vi "GFL_Get_Single_Fault_Snapshot.vi"(0 "GEA2 Reference In":refnum<k24>, 5 "Standalone?":bool, 7 "Snapshot Selection":T2, 11 "Error In":errorcluster) -> (4 "GEA2 Reference Out":refnum<k24>, 6 "Fault Snapshots":T1, 15 "Error Out":errorcluster)   [LabVIEW 2016]
uses:
  subVIs/Snap_Selection.ctl
  C:/Automation/DLLs/PC Dot Net/GeaCommunication.dll
  subVIs/Snap_Input.ctl
  Common/LabVIEW GEA2 Toolkit/LabVIEW_GEA2_Toolkit.lvlibp/type defs/Source_Destination.ctl
  Common/LabVIEW GEA2 Toolkit/LabVIEW_GEA2_Toolkit.lvlibp/type defs/ERD Read Data In.ctl
  Common/LabVIEW GEA2 Toolkit/LabVIEW_GEA2_Toolkit.lvlibp/type defs/Data Type.ctl
  Common/LabVIEW GEA2 Toolkit/LabVIEW_GEA2_Toolkit.lvlibp
panel:
  out "ERD Number":string
  out "ERD Data":string
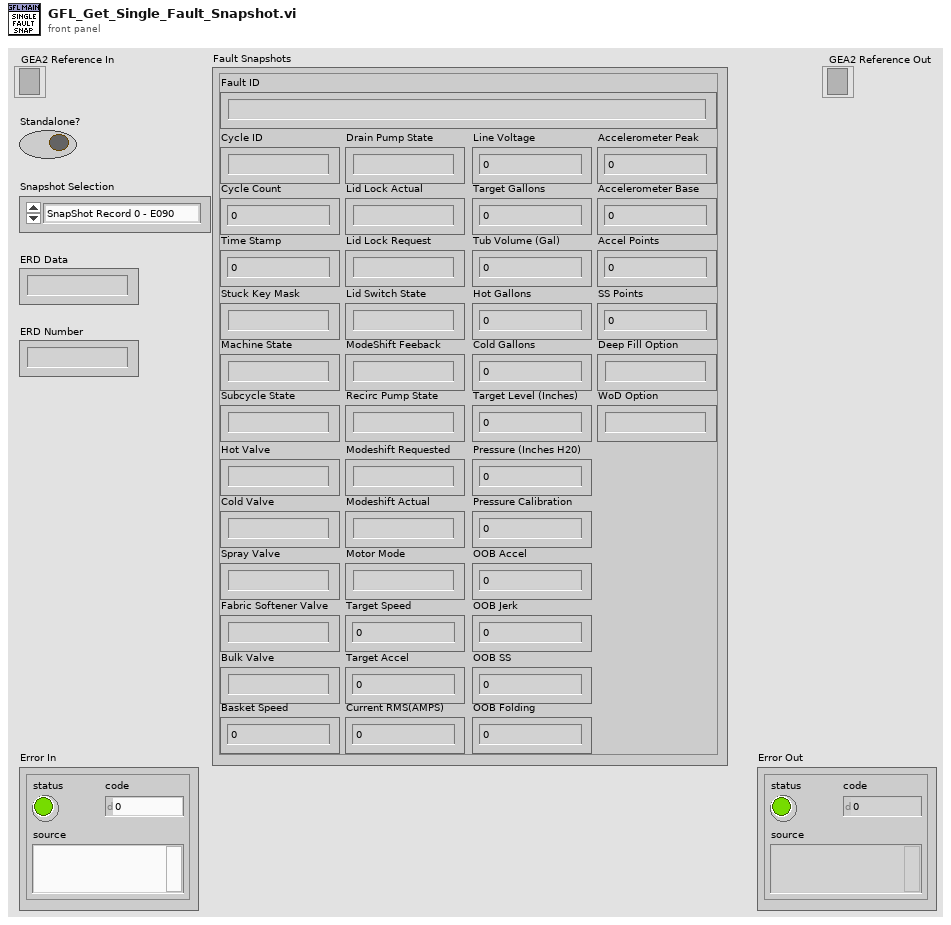
[diagram p1: front panel]
types:
  T1 = typedef "Snap_Input.ctl" = cluster{"Fault ID":string, "Cycle Count":u32, "Cycle ID":string, "Time Stamp":u32, "Stuck Key Mask":string, "Machine State":string, "Subcycle State":string, "Hot Valve":string, "Cold Valve":string, "Spray Valve":string, "Fabric Softener Valve":string, "Bulk Valve":string, "Drain Pump State":string, "Lid Lock Actual":string, "Lid Lock Request":string, "Lid Switch State":string, "ModeShift Feeback":string, "Recirc Pump State":string, "Modeshift Requested":string, "Modeshift Actual":string, "Motor Mode":string, "Target Speed":u16, "Target Accel":u16, "Current RMS(AMPS)":dbl, "Line Voltage":dbl, "Target Gallons":dbl, "Tub Volume (Gal)":dbl, "Hot Gallons":dbl, "Cold Gallons":dbl, "Target Level (Inches)":dbl, "Pressure (Inches H20) ":dbl, "Pressure Calibration":dbl, "OOB Accel":i32, "OOB Jerk":i32, "OOB SS":i32, "OOB Folding":i32, "Accelerometer Peak":i16, "Accelerometer Base":i16, "Accel Points":u8, "SS Points":u8, "Deep Fill Option":string, "WoD Option":string, "Basket Speed":u16}
  T2 = typedef "Snap_Selection.ctl" = enum16{"SnapShot Record 0 - E090", "Snapshot Record 1 - E091", "Snapshot Record 2 - E092"}
  T3 = typedef "LabVIEW_GEA2_Toolkit.lvlibp/Source_Destination.ctl" = cluster{"Source":u8, "Destination":u8}
  T4 = typedef "LabVIEW_GEA2_Toolkit.lvlibp/ERD Read Data In.ctl" = cluster{"ERD Number":u16, "Data Type":T5}
  T5 = typedef "LabVIEW_GEA2_Toolkit.lvlibp/Data Type.ctl" = enum16{"string", "boolean", "uint8_t", "uint16_t", "uint32_t", "uint64_t", "int8_t", "int16_t", "int32_t", "int64_t"}
  T6 = typedef "LabVIEW_GEA2_Toolkit.lvlibp/ERD Read Data Out.ctl" = cluster{"ERD Number":u16, "Data":string}
  T7 = cluster{"ERD Data Out[0]":T6, "ERD Data Out[1]":T6, "ERD Data Out[2]":T6, "ERD Data Out[3]":T6, "ERD Data Out[4]":T6, "ERD Data Out[5]":T6, "ERD Data Out[6]":T6, "ERD Data Out[7]":T6, "ERD Data Out[8]":T6}
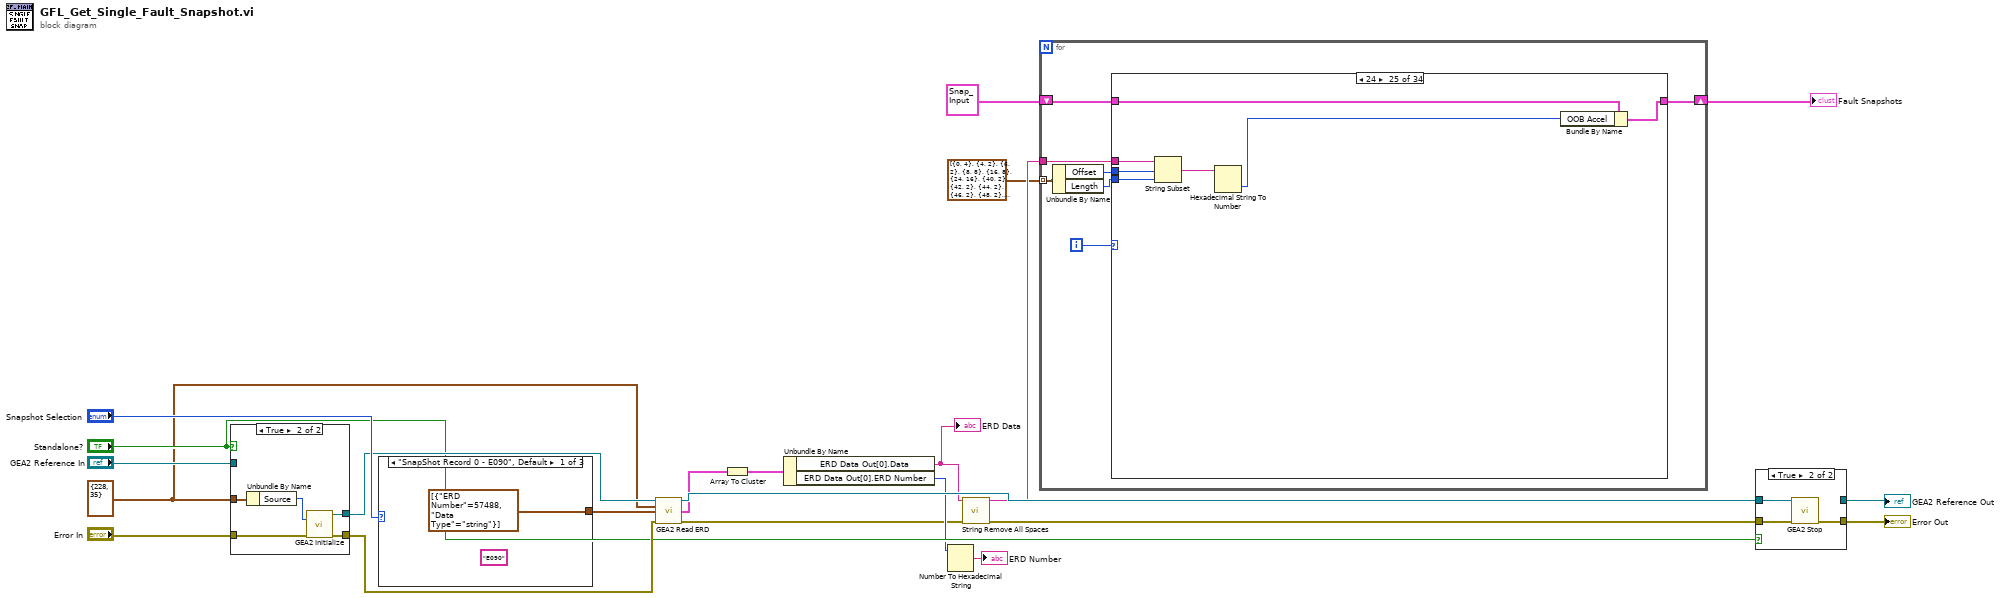
[diagram p0: block diagram]
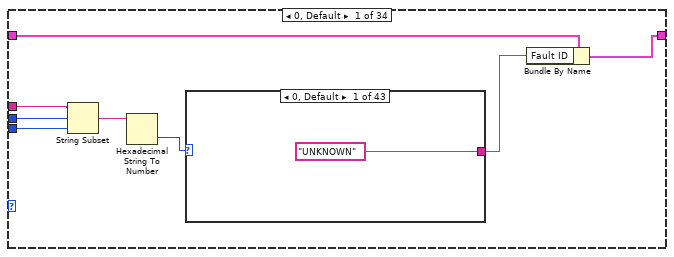
[diagram p2: hidden frame]
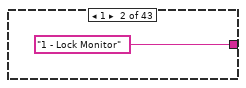
[diagram p3: hidden frame]
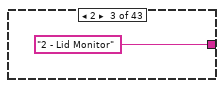
[diagram p4: hidden frame]
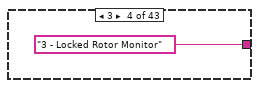
[diagram p5: hidden frame]
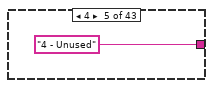
[diagram p6: hidden frame]
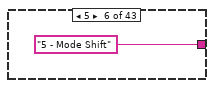
[diagram p7: hidden frame]
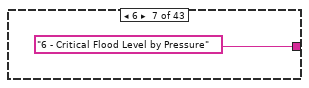
[diagram p8: hidden frame]
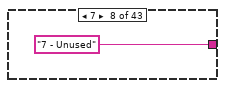
[diagram p9: hidden frame]
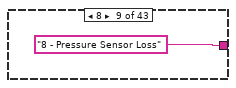
[diagram p10: hidden frame]
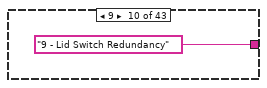
[diagram p11: hidden frame]
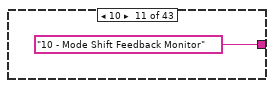
[diagram p12: hidden frame]
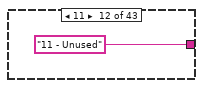
[diagram p13: hidden frame]
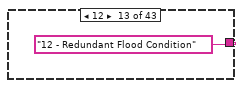
[diagram p14: hidden frame]
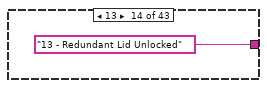
[diagram p15: hidden frame]
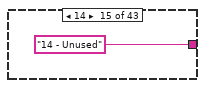
[diagram p16: hidden frame]
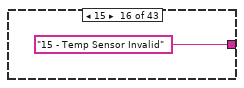
[diagram p17: hidden frame]
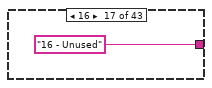
[diagram p18: hidden frame]
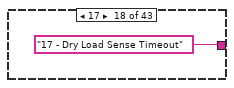
[diagram p19: hidden frame]
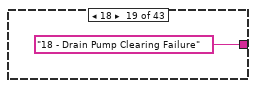
[diagram p20: hidden frame]
diagram:
  w13 = T3 {"Source"=228, "Destination"=35} ("GEA Inputs")
  n1 = case shown="True" "Standalone?" {
    tunnel: "Error In" -> [w23 w29]
    tunnel: [w23 w28] -> w17
    tunnel: "GEA2 Reference In" -> [w24 _]
    tunnel: [w24 w27] -> w18
    tunnel: w13 -> [_ w25]
    frame False {
    }
    frame True {
      n2 = Unbundle By Name(w25) -> ("Source"=w26:u8)
      n3 = call "GEA2 Initialize.vi"("Source Address"=w26, "error in"=w29) -> ("GEA2 Reference Out"=w27:refnum<k24>, "error out"=w28:errorcluster)  [unwired: 11 in, 1 out]
    }
  }
  n4 = case shown="\"SnapShot Record 0 - E090\", Default" "Snapshot Selection" {
    tunnel: [T4[] [{"ERD Number"=57488, "Data Type"=enum."string"}] ("Read ERD List") T4[] [{"ERD Number"=57489, "Data Type"=enum."string"}] ("Read ERD List") T4[] [{"ERD Number"=57490, "Data Type"=enum."string"}] ("Read ERD List")] -> w21
    frame "SnapShot Record 0 - E090", Default {
      (unwired) "E090"
    }
    frame "Snapshot Record 1 - E091" {
      (unwired) "E091"
    }
    frame "Snapshot Record 2 - E092" {
      (unwired) "E092"
    }
  }
  n5 = call "GEA2 Read ERD.vi"("GEA2 Reference In"=w18, "GEA Inputs"=w13, "Read ERD List"=w21, "Error In"=w17) -> ("GEA2 Reference Out"=w16:refnum<k24>, "ERD Data Out"=w12:T6[], "Error Out"=w7:errorcluster)  [unwired: 8 in, 1 out]
  n6 = Array To Cluster(array=w12) -> (cluster=w11:T7)
  n7 = Unbundle By Name(w11) -> ("ERD Data Out[0].Data"=w8:string, "ERD Data Out[0].ERD Number"=w10:u16)
  "ERD Data" <- w8
  n8 = Number To Hexadecimal String(2:w10) -> (0:→"ERD Number":string)  [unwired: 1 in]
  n9 = call "String Remove All Spaces.vi"("Input String"=w8, "error in (no error)"=w7) -> ("Spaces Removed"=w4:string, "error out"=w6:errorcluster)  [unwired: 12 in]
  n10 = for {
    tunnel: w4 -> [w39]
    shift-right: [w37] -> w1
    shift-left: T1 {"Fault ID"="", "Cycle Count"=0, "Cycle ID"="", "Time Stamp"=0, "Stuck Key Mask"="", "Machine State"="", "Subcycle State"="", "Hot Valve"="", "Cold Valve"="", "Spray Valve"="", "Fabric Softener Valve"="", "Bulk Valve"="", "Drain Pump State"="", "Lid Lock Actual"="", "Lid Lock Request"="", "Lid Switch State"="", "ModeShift Feeback"="", "Recirc Pump State"="", "Modeshift Requested"="", "Modeshift Actual"="", "Motor Mode"="", "Target Speed"=0, "Target Accel"=0, "Current RMS(AMPS)"=0.0, "Line Voltage"=0.0, "Target Gallons"=0.0, "Tub Volume (Gal)"=0.0, "Hot Gallons"=0.0, "Cold Gallons"=0.0, "Target Level (Inches)"=0.0, "Pressure (Inches H20) "=0.0, "Pressure Calibration"=0.0, "OOB Accel"=0, "OOB Jerk"=0, "OOB SS"=0, "OOB Folding"=0, "Accelerometer Peak"=0, "Accelerometer Base"=0, "Accel Points"=0, "SS Points"=0, "Deep Fill Option"="", "WoD Option"="", "Basket Speed"=0} ("input cluster") -> [w38]
    tunnel: cluster{"Offset":i32, "Length":i32}[] [{"Offset"=0, "Length"=4}, {"Offset"=4, "Length"=2}, {"Offset"=6, "Length"=2}, {"Offset"=8, "Length"=8}, {"Offset"=16, "Length"=8}, {"Offset"=24, "Length"=16}, {"Offset"=40, "Length"=2}, {"Offset"=42, "Length"=2}, {"Offset"=44, "Length"=2}, {"Offset"=46, "Length"=2}, {"Offset"=48, "Length"=2}, {"Offset"=50, "Length"=2}, {"Offset"=52, "Length"=4}, {"Offset"=56, "Length"=4}, {"Offset"=60, "Length"=4}, {"Offset"=64, "Length"=4}, {"Offset"=68, "Length"=4}, {"Offset"=72, "Length"=4}, {"Offset"=76, "Length"=4}, {"Offset"=80, "Length"=4}, {"Offset"=84, "Length"=4}, {"Offset"=88, "Length"=8}, {"Offset"=96, "Length"=8}, {"Offset"=104, "Length"=8}, {"Offset"=112, "Length"=8}, {"Offset"=120, "Length"=8}, {"Offset"=128, "Length"=8}, {"Offset"=136, "Length"=8}, {"Offset"=144, "Length"=4}, {"Offset"=148, "Length"=4}, {"Offset"=152, "Length"=2}, {"Offset"=154, "Length"=2}, {"Offset"=156, "Length"=2}, {"Offset"=158, "Length"=2}] -> [w34] mode=indexing
    i -> [w36]
    n11 = Unbundle By Name(w34) -> ("Offset"=w35:i32, "Length"=w33:i32)
    n12 = case shown="24" w36 {
      tunnel: w39 -> [w46 w98 _ w143 w152 w158 w181 w201 w228 w264 w287 w300 w315 w323 w331 w341 w351 w361 w371 w381 w391 w401 w411 w421 w428 w435 w442 w449 w456 w463 w470 w477 w485 w489]
      tunnel: w35 -> [w45 w97 _ w142 w151 w157 w180 w200 w227 w263 w286 w299 w314 w322 w330 w340 w350 w360 w370 w380 w390 w400 w410 w420 w427 w434 w441 w448 w455 w462 w469 w476 w484 w488]
      tunnel: w33 -> [w44 w96 _ w141 w150 w156 w179 w199 w226 w262 w285 w298 w313 w321 w329 w339 w349 w359 w369 w379 w389 w399 w409 w419 w426 w433 w440 w447 w454 w461 w468 w475 w483 w487]
      tunnel: w38 -> [w47 w95 w138 w145 w149 w160 w183 w198 w230 w266 w289 w302 w317 w325 w333 w343 w353 w363 w373 w383 w393 w403 w413 w423 w430 w437 w444 w451 w458 w465 w472 w479 w481 w491]
      tunnel: [w43 w94 w138 w144 w148 w159 w182 w197 w229 w265 w288 w301 w316 w324 w332 w342 w352 w362 w372 w382 w392 w402 w412 w422 w429 w436 w443 w450 w457 w464 w471 w478 w480 w490] -> w37
      frame 0, Default {
        n13 = String Subset(string=w46, offset (0)=w45, length (rest)=w44) -> (substring=w42:string)
        n14 = Hexadecimal String To Number(string=w42) -> (number=w41:u32)  [unwired: 2 in, 1 out]
        n15 = case shown="0, Default" w41 {
          tunnel: ["UNKNOWN" "1 - Lock Monitor" "2 - Lid Monitor" "3 - Locked Rotor Monitor" "4 - Unused" "5 - Mode Shift" "6 - Critical Flood Level by Pressure" "7 - Unused" "8 - Pressure Sensor Loss" "9 - Lid Switch Redundancy" "10 - Mode Shift Feedback Monitor" "11 - Unused" "12 - Redundant Flood Condition" "13 - Redundant Lid Unlocked" "14 - Unused" "15 - Temp Sensor Invalid" "16 - Unused" "17 - Dry Load Sense Timeout" "18 - Drain Pump Clearing Failure" "19 - UI State Timeout" "20 - Critical Flood Level by Gallons" "21 - Unused " "22 - OOB during dry load sense" "23 - Critical Lid Lock Failure: Can't Lock" "24 - Lid Logic Failure" "25 - Pressure Sensor Dropout" "26 - OOB Redistribution" "27 - Water Accessibility" "28 - ADC Knob Feedback Invalid" "29 - Suds Lock Abatement Failure" "30 - Stuck Button Fault" "31 - OOB Fallback In Final Spin" "32 - Critical Lid Lock Failure: Can't Unlock" "100 - Accelerometer Communication Error" "101 - Max Fill Pressure" "102 - Clock Monitor" "103 - LidLock Failure" "104 - Adaptive Drain" "105 - Max Fill Volume" "106 - Target Spin Speed Timeout" "107 - Target Spin Speed Dropout" "108 - UI-MC Heartbeat Communication Failure" "109 - Event Sequence Buffer Overrun"] -> w40
          frame 0, Default {
          }
          frame 1 {
          }
          frame 2 {
          }
          frame 3 {
          }
          frame 4 {
          }
          frame 5 {
          }
          frame 6 {
          }
          frame 7 {
          }
          frame 8 {
          }
          frame 9 {
          }
          frame 10 {
          }
          frame 11 {
          }
          frame 12 {
          }
          frame 13 {
          }
          frame 14 {
          }
          frame 15 {
          }
          frame 16 {
          }
          frame 17 {
          }
          frame 18 {
          }
          frame 19 {
          }
          frame 20 {
          }
          frame 21 {
          }
          frame 22 {
          }
          frame 23 {
          }
          frame 24 {
          }
          frame 25 {
          }
          frame 26 {
          }
          frame 27 {
          }
          frame 28 {
          }
          frame 29 {
          }
          frame 30 {
          }
          frame 31 {
          }
          frame 32 {
          }
          frame 100 {
          }
          frame 101 {
          }
          frame 102 {
          }
          frame 103 {
          }
          frame 104 {
          }
          frame 105 {
          }
          frame 106 {
          }
          frame 107 {
          }
          frame 108 {
          }
          frame 109 {
          }
        }
        n16 = Bundle By Name(cluster=w47, "Fault ID"=w40) -> (w43:T1)
      }
      frame 1 {
        n17 = String Subset(string=w98, offset (0)=w97, length (rest)=w96) -> (substring=w93:string)
        n18 = Hexadecimal String To Number(string=w93) -> (number=w92:u32)  [unwired: 2 in, 1 out]
        n19 = case shown="0, Default" w92 {
          tunnel: ["0 - NotDefined" "1 - BasketClean" "2 - DrainAndSpin" "3 - QuickRinse" "4 - BulkyItems" "5 - Sanitize" "6 - TowelsSheets" "8 - Normal_Mixedload" "9 - Whites" "10 - DarkColors" "11 - Jeans" "12 - HandWash" "13 - Delicates" "14 - SpeedWash" "15 - HeavyDuty" "16 - Allergen" "17 - PowerClean" "18 - RinseSpin" "19 - SingleItemWash" "20 - Colors" "21 - ColdWash" "22 - WaterOnDemand" "23 - NotUsed_Start" "127 - NotUsed_End" "128 - Cottons" "129 - EasyCare" "130 - ActiveWear" "131 - TimedDry" "132 - DeWrinkle" "133 - QuickAirFluff" "134 - SteamRefresh" "135 - SteamDewrinkle" "136 - SpeedDry" "137 - Mixed" "138 - Quickdry" "139 - Casuals" "140 - Warmup" "141 - EnergySaver" "142 - Antibacterial"] -> w91
          frame 0, Default {
          }
          frame 1 {
          }
          frame 2 {
          }
          frame 3 {
          }
          frame 4 {
          }
          frame 5 {
          }
          frame 6 {
          }
          frame 8 {
          }
          frame 9 {
          }
          frame 10 {
          }
          frame 11 {
          }
          frame 12 {
          }
          frame 13 {
          }
          frame 14 {
          }
          frame 15 {
          }
          frame 16 {
          }
          frame 17 {
          }
          frame 18 {
          }
          frame 19 {
          }
          frame 20 {
          }
          frame 21 {
          }
          frame 22 {
          }
          frame 23 {
          }
          frame 127 {
          }
          frame 128 {
          }
          frame 129 {
          }
          frame 130 {
          }
          frame 131 {
          }
          frame 132 {
          }
          frame 133 {
          }
          frame 134 {
          }
          frame 135 {
          }
          frame 136 {
          }
          frame 137 {
          }
          frame 138 {
          }
          frame 139 {
          }
          frame 140 {
          }
          frame 141 {
          }
          frame 142 {
          }
        }
        n20 = Bundle By Name(cluster=w95, "Cycle ID"=w91) -> (w94:T1)
      }
      frame 2 {
        # "Paddding"
      }
      frame 3 {
        n21 = String Subset(string=w143, offset (0)=w142, length (rest)=w141) -> (substring=w140:string)
        n22 = Hexadecimal String To Number(string=w140) -> (number=w139:u32)  [unwired: 2 in, 1 out]
        n23 = Bundle By Name(cluster=w145, "Cycle Count"=w139) -> (w144:T1)
      }
      frame 4 {
        n24 = String Subset(string=w152, offset (0)=w151, length (rest)=w150) -> (substring=w147:string)
        n25 = Hexadecimal String To Number(string=w147) -> (number=w146:u32)  [unwired: 2 in, 1 out]
        n26 = Bundle By Name(cluster=w149, "Time Stamp"=w146) -> (w148:T1)
      }
      frame 5 {
        (unwired) ""
        n27 = String Subset(string=w158, offset (0)=w157, length (rest)=w156) -> (substring=w155:string)
        n28 = Hexadecimal String To Number(string=w155) -> (number=w154:u32)  [unwired: 2 in, 1 out]
        n29 = case shown="0, Default" w154 {
          tunnel: ["No Stuck Key" "Smart Dispense" "Delay Wash" "Extra Rinse" "Mycycle" "Spin Button" "Deep Rinse" "Soil Button" "Auto Soak" "Temp Button" "Warm Rinse" "Deep Fill" "Water on Demand" "Power Button" "Start Button"] -> w153
          frame 0, Default {
          }
          frame 1 {
          }
          frame 2 {
          }
          frame 4 {
          }
          frame 8 {
          }
          frame 16 {
          }
          frame 32 {
          }
          frame 64 {
          }
          frame 128 {
          }
          frame 256 {
          }
          frame 512 {
          }
          frame 1024 {
          }
          frame 2048 {
          }
          frame 4096 {
          }
          frame 8192 {
          }
        }
        n30 = Bundle By Name(cluster=w160, "Stuck Key Mask"=w153) -> (w159:T1)
      }
      frame 6 {
        n31 = String Subset(string=w181, offset (0)=w180, length (rest)=w179) -> (substring=w178:string)
        n32 = Hexadecimal String To Number(string=w178) -> (number=w177:u32)  [unwired: 2 in, 1 out]
        n33 = case shown="128" w177 {
          tunnel: ["IDLE" "STANDBY" "RUN" "PAUSE" "EOC" "DSM DELAY RUN" "DELAY RUN" "DELAY PAUSE" "DRAIN TIMEOUT" "CLEAN SPEAK"] -> w176
          frame 0, Default {
          }
          frame 1 {
          }
          frame 2 {
          }
          frame 3 {
          }
          frame 4 {
          }
          frame 5 {
          }
          frame 6 {
          }
          frame 7 {
          }
          frame 8 {
          }
          frame 128 {
          }
        }
        n34 = Bundle By Name(cluster=w183, "Machine State"=w176) -> (w182:T1)
      }
      frame 7 {
        n35 = String Subset(string=w201, offset (0)=w200, length (rest)=w199) -> (substring=w196:string)
        n36 = Hexadecimal String To Number(string=w196) -> (number=w195:u32)  [unwired: 2 in, 1 out]
        n37 = case shown="0, Default" w195 {
          tunnel: ["NONE" "FILL" "SOAK" "WASH" "RINSE" "SPIN" "DRAIN" "EXTRA SPIN" "EXTRA RINSE" "TUMBLE" "LOAD SIZE"] -> w194
          frame 0, Default {
          }
          frame 1 {
          }
          frame 2 {
          }
          frame 3 {
          }
          frame 4 {
          }
          frame 5 {
          }
          frame 6 {
          }
          frame 7 {
          }
          frame 8 {
          }
          frame 9 {
          }
          frame 10 {
          }
        }
        n38 = Bundle By Name(cluster=w198, "Subcycle State"=w194) -> (w197:T1)
      }
      frame 8 {
        n39 = String Subset(string=w228, offset (0)=w227, length (rest)=w226) -> (substring=w224:string)
        n40 = Hexadecimal String To Number(string=w224) -> (number=w225:u32)  [unwired: 2 in, 1 out]
        n41 = Number To Boolean Array(number=w225) -> (Boolean array=w223:bool[])
        n42 = Index Array(array=w223) -> (element #1=w222:bool, element #2=w220:bool, element #3=w219:bool, element #4=w218:bool, element #5=w217:bool)  [unwired: 5 in]
        n43 = case shown="False" w222 {
          tunnel: ["OFF" "ON"] -> w221
          frame False {
          }
          frame True {
          }
        }
        n44 = case shown="False" w220 {
          tunnel: ["OFF" "ON"] -> w216
          frame False {
          }
          frame True {
          }
        }
        n45 = case shown="False" w219 {
          tunnel: ["OFF" "ON"] -> w215
          frame False {
          }
          frame True {
          }
        }
        n46 = case shown="False" w218 {
          tunnel: ["OFF" "ON"] -> w214
          frame False {
          }
          frame True {
          }
        }
        n47 = case shown="False" w217 {
          tunnel: ["OFF" "ON"] -> w213
          frame False {
          }
          frame True {
          }
        }
        n48 = Bundle By Name(cluster=w230, "Hot Valve"=w221, "Cold Valve"=w216, "Spray Valve"=w215, "Fabric Softener Valve"=w214, "Bulk Valve"=w213) -> (w229:T1)
      }
      frame 9 {
        n49 = String Subset(string=w264, offset (0)=w263, length (rest)=w262) -> (substring=w261:string)
        n50 = Hexadecimal String To Number(string=w261) -> (number=w260:u32)  [unwired: 2 in, 1 out]
        n51 = Number To Boolean Array(number=w260) -> (Boolean array=w259:bool[])
        n52 = Index Array(array=w259) -> (element #1=w257:bool, element #2=w256:bool, element #3=w253:bool, element #4=w252:bool, element #5=w249:bool, element #6=w248:bool, element #7=w246:bool, element #8=w245:bool)  [unwired: 8 in]
        n53 = Boolean To (0,1)(Boolean=w246) -> (0, 1=w243:i16)
        n54 = Boolean To (0,1)(Boolean=w245) -> (0, 1=w244:i16)
        n55 = Add(x=w243, y=w244) -> (x+y=w242:i16)
        n56 = case shown="True" w249 {
          tunnel: ["AGITATE" "SPIN"] -> w250
          frame False {
          }
          frame True {
          }
        }
        n57 = case shown="True" w248 {
          tunnel: ["OFF" "ON"] -> w247
          frame False {
          }
          frame True {
          }
        }
        n58 = case shown="True" w257 {
          tunnel: ["OFF" "ON"] -> w258
          frame False {
          }
          frame True {
          }
        }
        n59 = case shown="True" w256 {
          tunnel: ["UNLOCKED" "LOCKED"] -> w255
          frame False {
          }
          frame True {
          }
        }
        n60 = case shown="True" w253 {
          tunnel: ["UNLOCKED" "LOCKED"] -> w254
          frame False {
          }
          frame True {
          }
        }
        n61 = case shown="True" w252 {
          tunnel: ["OPEN" "CLOSED"] -> w251
          frame False {
          }
          frame True {
          }
        }
        n62 = case shown="2" w242 {
          tunnel: ["UNKNOWN" "AGITATE" "SPIN"] -> w241
          frame 0, Default {
          }
          frame 1 {
          }
          frame 2 {
          }
        }
        n63 = Bundle By Name(cluster=w266, "Drain Pump State"=w258, "Lid Lock Actual"=w255, "Lid Lock Request"=w254, "Lid Switch State"=w251, "ModeShift Feeback"=w250, "Recirc Pump State"=w247, "Modeshift Requested"=w241) -> (w265:T1)
      }
      frame 10 {
        n64 = String Subset(string=w287, offset (0)=w286, length (rest)=w285) -> (substring=w284:string)
        n65 = Hexadecimal String To Number(string=w284) -> (number=w283:u32)  [unwired: 2 in, 1 out]
        n66 = case shown="4" w283 {
          tunnel: ["UNKNOWN" "AGITATE" "SPIN" "TRANS TO SPIN" "TRANS TO AGITATE"] -> w282
          frame 0, Default {
          }
          frame 1 {
          }
          frame 2 {
          }
          frame 3 {
          }
          frame 4 {
          }
        }
        n67 = Bundle By Name(cluster=w289, "Modeshift Actual"=w282) -> (w288:T1)
      }
      frame 11 {
        n68 = String Subset(string=w300, offset (0)=w299, length (rest)=w298) -> (substring=w297:string)
        n69 = Hexadecimal String To Number(string=w297) -> (number=w296:u32)  [unwired: 2 in, 1 out]
        n70 = case shown="0, Default" w296 {
          tunnel: ["CLOSED LOOP" "CLOSED LOOP ANGLE" "OPEN LOOP" "OPEN LOOP ANGLE" "COASTING" "BRAKING" "IDLE"] -> w295
          frame 0, Default {
          }
          frame 1 {
          }
          frame 2 {
          }
          frame 3 {
          }
          frame 4 {
          }
          frame 5 {
          }
          frame 6 {
          }
        }
        n71 = Bundle By Name(cluster=w302, "Motor Mode"=w295) -> (w301:T1)
      }
      frame 12 {
        n72 = String Subset(string=w315, offset (0)=w314, length (rest)=w313) -> (substring=w312:string)
        n73 = Hexadecimal String To Number(string=w312) -> (number=w311:u32)  [unwired: 2 in, 1 out]
        n74 = To Unsigned Word Integer(number=w311) -> (unsigned 16bit integer=w310:u16)
        n75 = Bundle By Name(cluster=w317, "Target Speed"=w310) -> (w316:T1)
      }
      frame 13 {
        n76 = String Subset(string=w323, offset (0)=w322, length (rest)=w321) -> (substring=w320:string)
        n77 = Hexadecimal String To Number(string=w320) -> (number=w319:u32)  [unwired: 2 in, 1 out]
        n78 = To Unsigned Word Integer(number=w319) -> (unsigned 16bit integer=w318:u16)
        n79 = Bundle By Name(cluster=w325, "Target Accel"=w318) -> (w324:T1)
      }
      frame 14 {
        n80 = String Subset(string=w331, offset (0)=w330, length (rest)=w329) -> (substring=w328:string)
        n81 = Hexadecimal String To Number(string=w328) -> (number=w327:u32)  [unwired: 2 in, 1 out]
        n82 = To Unsigned Word Integer(number=w327) -> (unsigned 16bit integer=w326:u16)
        n83 = Bundle By Name(cluster=w333, "Basket Speed"=w326) -> (w332:T1)
      }
      frame 15 {
        n84 = String Subset(string=w341, offset (0)=w340, length (rest)=w339) -> (substring=w338:string)
        n85 = Hexadecimal String To Number(string=w338) -> (number=w337:u32)  [unwired: 2 in, 1 out]
        n86 = To Double Precision Float(number=w337) -> (double precision float=w336:dbl)
        n87 = Divide(x=w336, y=1024.0) -> (x/y=w334:dbl)
        n88 = Bundle By Name(cluster=w343, "Current RMS(AMPS)"=w334) -> (w342:T1)
      }
      frame 16 {
        n89 = String Subset(string=w351, offset (0)=w350, length (rest)=w349) -> (substring=w348:string)
        n90 = Hexadecimal String To Number(string=w348) -> (number=w347:u32)  [unwired: 2 in, 1 out]
        n91 = To Double Precision Float(number=w347) -> (double precision float=w346:dbl)
        n92 = Divide(x=w346, y=32.0) -> (x/y=w344:dbl)
        n93 = Bundle By Name(cluster=w353, "Line Voltage"=w344) -> (w352:T1)
      }
      frame 17 {
        n94 = String Subset(string=w361, offset (0)=w360, length (rest)=w359) -> (substring=w358:string)
        n95 = Hexadecimal String To Number(string=w358) -> (number=w355:u32)  [unwired: 2 in, 1 out]
        n96 = To Double Precision Float(number=w355) -> (double precision float=w357:dbl)
        n97 = Divide(x=w357, y=100.0) -> (x/y=w354:dbl)
        n98 = Bundle By Name(cluster=w363, "Target Gallons"=w354) -> (w362:T1)
      }
      frame 18 {
        n99 = String Subset(string=w371, offset (0)=w370, length (rest)=w369) -> (substring=w368:string)
        n100 = Hexadecimal String To Number(string=w368) -> (number=w365:u32)  [unwired: 2 in, 1 out]
        n101 = To Double Precision Float(number=w365) -> (double precision float=w367:dbl)
        n102 = Divide(x=w367, y=100.0) -> (x/y=w364:dbl)
        n103 = Bundle By Name(cluster=w373, "Tub Volume (Gal)"=w364) -> (w372:T1)
      }
      frame 19 {
        n104 = String Subset(string=w381, offset (0)=w380, length (rest)=w379) -> (substring=w378:string)
        n105 = Hexadecimal String To Number(string=w378) -> (number=w375:u32)  [unwired: 2 in, 1 out]
        n106 = To Double Precision Float(number=w375) -> (double precision float=w377:dbl)
        n107 = Divide(x=w377, y=100.0) -> (x/y=w374:dbl)
        n108 = Bundle By Name(cluster=w383, "Hot Gallons"=w374) -> (w382:T1)
      }
      frame 20 {
        n109 = String Subset(string=w391, offset (0)=w390, length (rest)=w389) -> (substring=w388:string)
        n110 = Hexadecimal String To Number(string=w388) -> (number=w385:u32)  [unwired: 2 in, 1 out]
        n111 = To Double Precision Float(number=w385) -> (double precision float=w387:dbl)
        n112 = Divide(x=w387, y=100.0) -> (x/y=w384:dbl)
        n113 = Bundle By Name(cluster=w393, "Cold Gallons"=w384) -> (w392:T1)
      }
      frame 21 {
        n114 = String Subset(string=w401, offset (0)=w400, length (rest)=w399) -> (substring=w398:string)
        n115 = Hexadecimal String To Number(string=w398) -> (number=w395:u32)  [unwired: 2 in, 1 out]
        n116 = To Double Precision Float(number=w395) -> (double precision float=w397:dbl)
        n117 = Divide(x=w397, y=1000.0) -> (x/y=w394:dbl)
        n118 = Bundle By Name(cluster=w403, "Target Level (Inches)"=w394) -> (w402:T1)
      }
      frame 22 {
        n119 = String Subset(string=w411, offset (0)=w410, length (rest)=w409) -> (substring=w408:string)
        n120 = Hexadecimal String To Number(string=w408) -> (number=w405:u32)  [unwired: 2 in, 1 out]
        n121 = To Double Precision Float(number=w405) -> (double precision float=w407:dbl)
        n122 = Divide(x=w407, y=1000.0) -> (x/y=w404:dbl)
        n123 = Bundle By Name(cluster=w413, "Pressure (Inches H20)"=w404) -> (w412:T1)
      }
      frame 23 {
        n124 = String Subset(string=w421, offset (0)=w420, length (rest)=w419) -> (substring=w418:string)
        n125 = Hexadecimal String To Number(string=w418) -> (number=w415:u32)  [unwired: 2 in, 1 out]
        n126 = To Double Precision Float(number=w415) -> (double precision float=w417:dbl)
        n127 = Divide(x=w417, y=1000.0) -> (x/y=w414:dbl)
        n128 = Bundle By Name(cluster=w423, "Pressure Calibration"=w414) -> (w422:T1)
      }
      frame 24 {
        n129 = String Subset(string=w428, offset (0)=w427, length (rest)=w426) -> (substring=w425:string)
        n130 = Hexadecimal String To Number(string=w425) -> (number=w424:u32)  [unwired: 2 in, 1 out]
        n131 = Bundle By Name(cluster=w430, "OOB Accel"=w424) -> (w429:T1)
      }
      frame 25 {
        n132 = String Subset(string=w435, offset (0)=w434, length (rest)=w433) -> (substring=w432:string)
        n133 = Hexadecimal String To Number(string=w432) -> (number=w431:u32)  [unwired: 2 in, 1 out]
        n134 = Bundle By Name(cluster=w437, "OOB Jerk"=w431) -> (w436:T1)
      }
      frame 26 {
        n135 = String Subset(string=w442, offset (0)=w441, length (rest)=w440) -> (substring=w439:string)
        n136 = Hexadecimal String To Number(string=w439) -> (number=w438:u32)  [unwired: 2 in, 1 out]
        n137 = Bundle By Name(cluster=w444, "OOB SS"=w438) -> (w443:T1)
      }
      frame 27 {
        n138 = String Subset(string=w449, offset (0)=w448, length (rest)=w447) -> (substring=w446:string)
        n139 = Hexadecimal String To Number(string=w446) -> (number=w445:u32)  [unwired: 2 in, 1 out]
        n140 = Bundle By Name(cluster=w451, "OOB Folding"=w445) -> (w450:T1)
      }
      frame 28 {
        n141 = String Subset(string=w456, offset (0)=w455, length (rest)=w454) -> (substring=w453:string)
        n142 = Hexadecimal String To Number(string=w453) -> (number=w452:u32)  [unwired: 2 in, 1 out]
        n143 = Bundle By Name(cluster=w458, "Accelerometer Peak"=w452) -> (w457:T1)
      }
      frame 29 {
        n144 = String Subset(string=w463, offset (0)=w462, length (rest)=w461) -> (substring=w460:string)
        n145 = Hexadecimal String To Number(string=w460) -> (number=w459:u32)  [unwired: 2 in, 1 out]
        n146 = Bundle By Name(cluster=w465, "Accelerometer Base"=w459) -> (w464:T1)
      }
      frame 30 {
        n147 = String Subset(string=w470, offset (0)=w469, length (rest)=w468) -> (substring=w467:string)
        n148 = Hexadecimal String To Number(string=w467) -> (number=w466:u32)  [unwired: 2 in, 1 out]
        n149 = Bundle By Name(cluster=w472, "Accel Points"=w466) -> (w471:T1)
      }
      frame 31 {
        n150 = String Subset(string=w477, offset (0)=w476, length (rest)=w475) -> (substring=w474:string)
        n151 = Hexadecimal String To Number(string=w474) -> (number=w473:u32)  [unwired: 2 in, 1 out]
        n152 = Bundle By Name(cluster=w479, "SS Points"=w473) -> (w478:T1)
      }
      frame 32 {
        n153 = String Subset(string=w485, offset (0)=w484, length (rest)=w483) -> (substring=w482:string)
        n154 = Bundle By Name(cluster=w481, "Deep Fill Option"=w482) -> (w480:T1)
      }
      frame 33 {
        n155 = String Subset(string=w489, offset (0)=w488, length (rest)=w487) -> (substring=w486:string)
        n156 = Bundle By Name(cluster=w491, "WoD Option"=w486) -> (w490:T1)
      }
    }
  }
  "Fault Snapshots" <- w1
  n157 = case shown="True" "Standalone?" {
    tunnel: [w492 w496] -> w5
    tunnel: w16 -> [w493 w495]
    tunnel: [w493 _] -> w15
    tunnel: w6 -> [w492 w494]
    frame False {
    }
    frame True {
      n158 = call "GEA2 Stop.vi"("GEA2 Reference In"=w495, "Error In"=w494) -> ("Error Out"=w496:errorcluster)  [unwired: 13 in]
    }
  }
  "GEA2 Reference Out" <- w15
  "Error Out" <- w5
